vi "ConvertProppelerCommand.vi"(1 "Propeller Command -5 to 5":dbl) -> (0 "Propeller Output PWM":dbl)   [LabVIEW 2011]
uses:
  <vilib>/NXT/Dual Mode Library/prims/inRangeAndCoerce/inRangeAndCoerce_float.vi
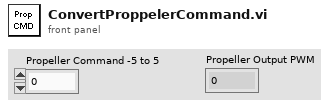
[diagram p1: front panel]
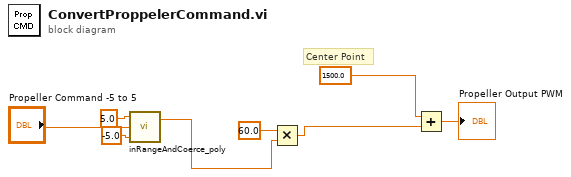
[diagram p0: block diagram]
diagram:
  # "Center Point"
  n1 = call-poly <vilib>:"inRangeAndCoerce_poly.vi"("lower limit"=-5.0, "x"="Propeller Command -5 to 5", "upper limit"=5.0) -> ("coerced(x)"=w3:dbl)  [unwired: 1 out]
  n2 = Multiply(x=60.0, y=w3) -> (x*y=w2:dbl)
  n3 = Add(x=1500.0 ("coerced(x)"), y=w2) -> (x+y=→"Propeller Output PWM":dbl)
